vi "krone.vi"(10 "Radius":sgl, 11 "Height":sgl) -> (0 "Fehler (Ausgang)":errorcluster, 3 "SceneObject (Ausgang)":refnum<vi>)   [LabVIEW 2014]
uses:
  <vilib>/picture/3D Picture Control/Object/Create Object (drawable).vi
  <vilib>/picture/3D Picture Control/NI_3D Picture Control.lvlib
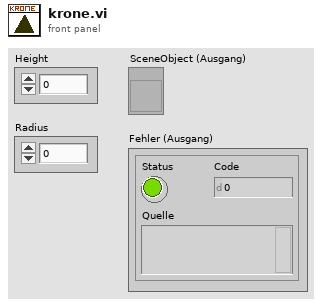
[diagram p1: front panel]
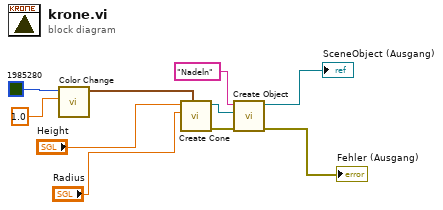
[diagram p0: block diagram]
diagram:
  n1 = call <vilib>:"Color Change.vi"("Alpha"=1.0, "Color"=u32 1985280) -> ("RGBA"=w8:cluster{"R":sgl, "G":sgl, "B":sgl, "A":sgl})  [unwired: 9 in]
  n2 = call <vilib>:"Create Cone.vi"("Color"=w8, "Radius"="Radius", "Height"="Height") -> ("error out"=w3:errorcluster, "New Cone Refnum"=w1:refnum<vi>)  [unwired: 7 in]
  n3 = call-poly <vilib>:"Create Object.vi"("error in (no error)"=w3, "Geometry"=w1, "Name"="Nadeln") -> ("error out"=→"Fehler (Ausgang)":errorcluster, "Scene:New Object"=→"SceneObject (Ausgang)":refnum<vi>)  [unwired: 7 in]
